vi "Config_SaveKeys.vi"(8 "error in (no error)":errorcluster, 9 "Configuration Save":T1={"General"={"Config.ini"=path "", "Default Logging Path"=path ""}, "Hardware"={"Measure Rate (1/s)"=0, "HP DMM VISA"="", "LS 335 VISA"="", "HP DM"={"Range"=enum."Autorange", "Autozero"=FALSE, "Display"=enum."3 1/2 Digit", "Blank LCD"=FALSE}}, "Operation"={"Operation Mode"=enum."Idle-Off", "Status"="", "NewLog?"=FALSE, "OvenWarn"=FALSE}}, 10 "Configuration Cluster":T1={"General"={"Config.ini"=path "", "Default Logging Path"=path ""}, "Hardware"={"Measure Rate (1/s)"=0, "HP DMM VISA"="", "LS 335 VISA"="", "HP DM"={"Range"=enum."Autorange", "Autozero"=FALSE, "Display"=enum."3 1/2 Digit", "Blank LCD"=FALSE}}, "Operation"={"Operation Mode"=enum."Idle-Off", "Status"="", "NewLog?"=FALSE, "OvenWarn"=FALSE}}, 11 "Config In":T3) -> (0 "error out":errorcluster, 2 "output cluster":T1={"General"={"Config.ini"=path "", "Default Logging Path"=path ""}, "Hardware"={"Measure Rate (1/s)"=0, "HP DMM VISA"="", "LS 335 VISA"="", "HP DM"={"Range"=enum."Autorange", "Autozero"=FALSE, "Display"=enum."3 1/2 Digit", "Blank LCD"=FALSE}}, "Operation"={"Operation Mode"=enum."Idle-Off", "Status"="", "NewLog?"=FALSE, "OvenWarn"=FALSE}}, 3 "refnum out":T3)   [LabVIEW 2021]
uses:
  <vilib>/Utility/config.llb/Config Data RefNum.ctl
  Config_Cluster.ctl
  Mode_Enum.ctl
  <vilib>/Utility/config.llb/Write Key (Path).vi
  <vilib>/Utility/config.llb/Write Key (String).vi
  <vilib>/Utility/config.llb/NI_LVConfig.lvlib
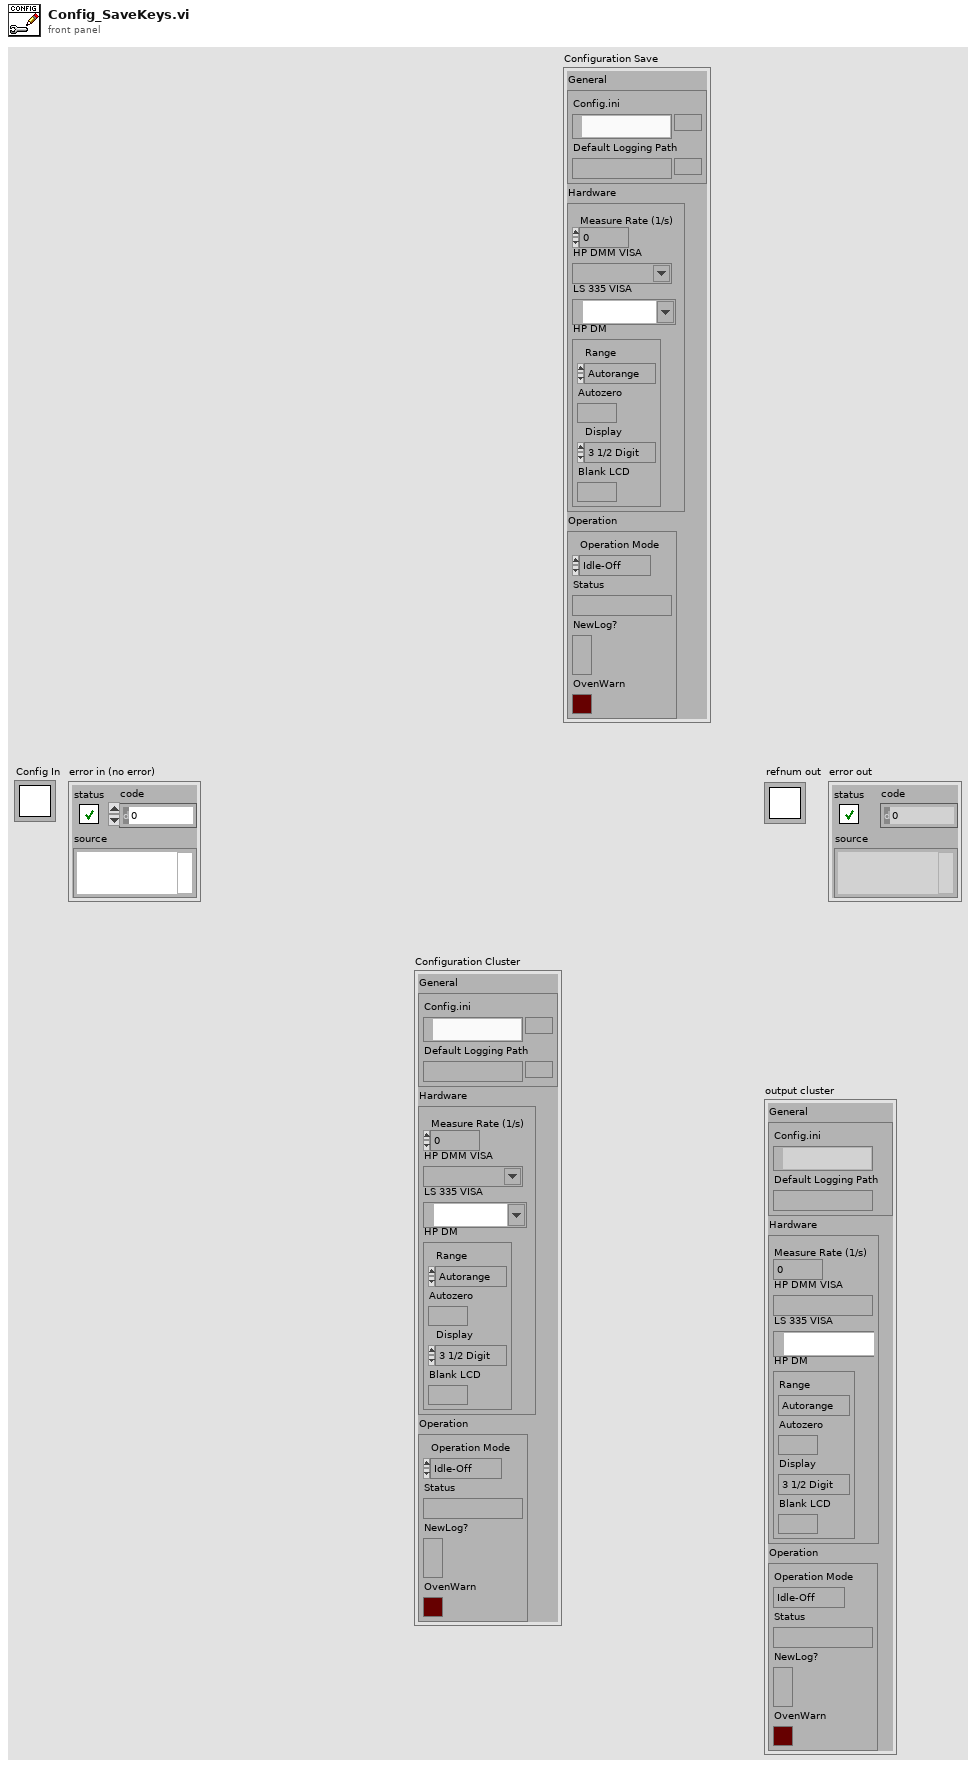
[diagram p1: front panel]
types:
  T1 = typedef "Config_Cluster.ctl" = cluster{"General":cluster{"Config.ini":path, "Default Logging Path":path}, "Hardware":cluster{"Measure Rate (1/s)":i32, "HP DMM VISA":refnum<visa-resource-name>, "LS 335 VISA":refnum<visa-resource-name>, "HP DM":cluster{"Range":enum16{"Autorange", "30mV", "300mV", "3V", "30V"}, "Autozero":bool, "Display":enum16{"3 1/2 Digit", "4 1/2 Digit", "5 1/2 Digit"}, "Blank LCD":bool}}, "Operation":cluster{"Operation Mode":T2, "Status":string, "NewLog?":bool, "OvenWarn":bool}}
  T2 = typedef "Mode_Enum.ctl" = enum16{"OvenNRDY", "Logging", "Idle-Off", "Idle"}
  T3 = typedef "NI_LVConfig.lvlib/Config Data RefNum.ctl" = refnum<k1>
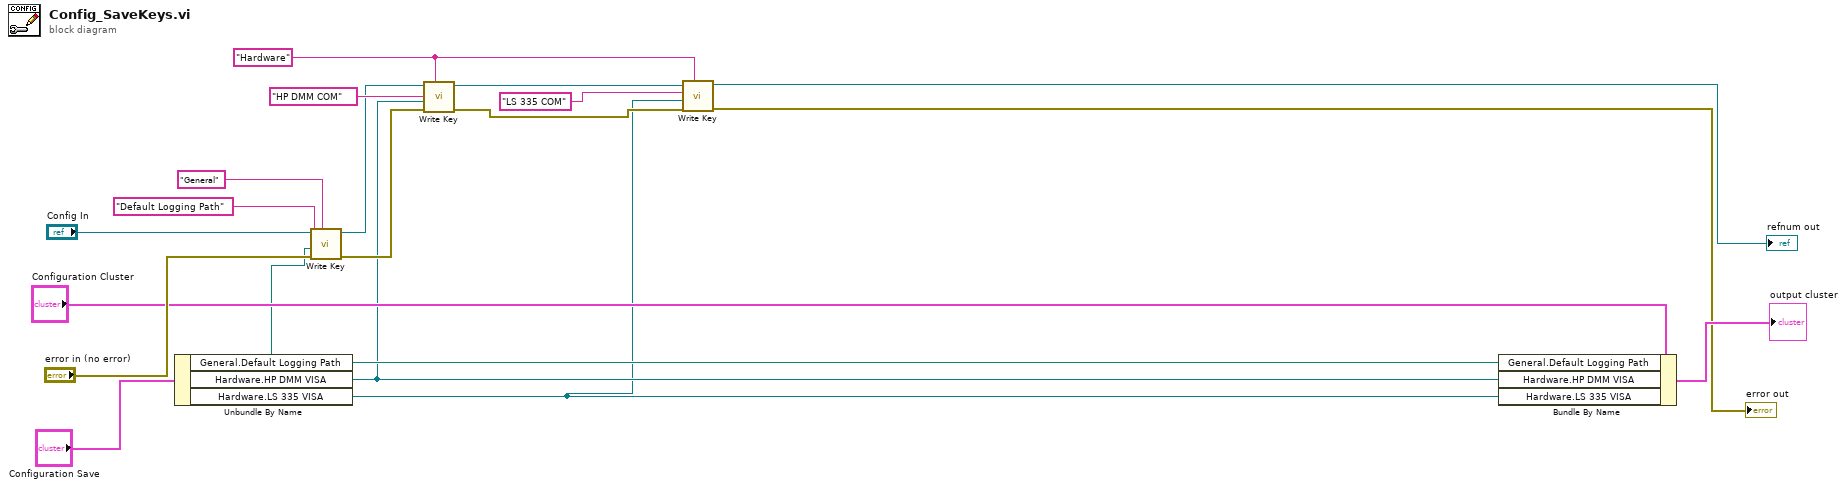
[diagram p0: block diagram]
diagram:
  w9 = "Hardware" ("section")
  n1 = Unbundle By Name("Configuration Save") -> ("General.Default Logging Path"=w3:path, "Hardware.HP DMM VISA"=w2:refnum<visa-resource-name>, "Hardware.LS 335 VISA"=w1:refnum<visa-resource-name>)
  n2 = call-poly <vilib>:"Write Key.vi"("section"="General", "error in (no error)"="error in (no error)", "value"=w3, "key"="Default Logging Path", "refnum"="Config In") -> ("error out"=w5:errorcluster, "refnum out"=w6:T3)  [unwired: 4 in, 1 out]
  n3 = call-poly <vilib>:"Write Key.vi"("section"=w9, "error in (no error)"=w5, "value"=w2, "key"="HP DMM COM", "refnum"=w6) -> ("error out"=w11:errorcluster, "refnum out"=w12:T3)  [unwired: 4 in, 1 out]
  n4 = call-poly <vilib>:"Write Key.vi"("section"=w9, "error in (no error)"=w11, "value"=w1, "key"="LS 335 COM", "refnum"=w12) -> ("error out"=→"error out":errorcluster, "refnum out"=→"refnum out":T3)  [unwired: 4 in, 1 out]
  n5 = Bundle By Name(cluster="Configuration Cluster", "General.Default Logging Path"=w3, "Hardware.HP DMM VISA"=w2, "Hardware.LS 335 VISA"=w1) -> (→"output cluster":T1)
